vi "Set scrollbar at start.vi"(8 "error in (no error)":errorcluster, 11 "Queue in":refnum<queue>) -> (0 "error out":errorcluster)   [LabVIEW 2013]
uses:
  Typedefs/Speed Viewer States enum.ctl
  Globals/gl_Time series viewer globals.vi
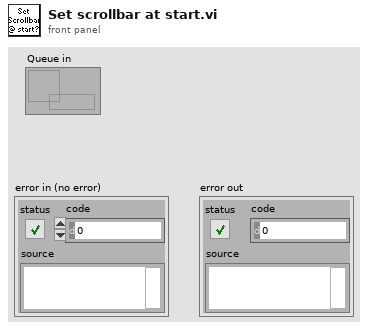
[diagram p1: front panel]
types:
  T1 = typedef "Timelapse viewer refs.ctl" = cluster{"This VI":refnum<vi>, "AVI Mode ind":refnum<vi>, "Play":refnum<vi>, "Stop":refnum<vi>, "Back":refnum<vi>, "Scrollbar":refnum<vi>, "Video length info":refnum<vi>, "Expected speed values":refnum<vi>, "Intensity":refnum<vi>, "Path":refnum<vi>, "Selection sliders":refnum<vi>, "Speed Graph ref":refnum<vi>, "Frame rate set (fps)":refnum<vi>}
  T2 = typedef "Speed Viewer States enum.ctl" = enum16{"Idle", "Initialise", "Playback", "Scroll bar event", "Speed cursor event", "Back to start", "Exit"}
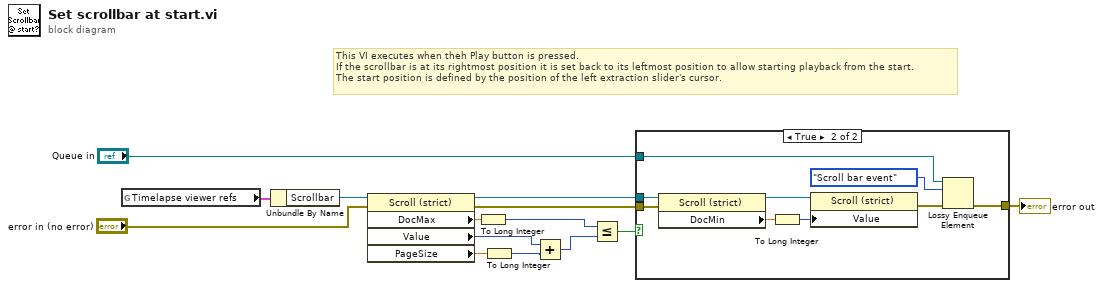
[diagram p0: block diagram]
diagram:
  # "This VI executes when theh Play button is pressed.\nIf the scrollbar is at its rightmost position it is set back to its leftmost position to allow starting playback from the start.\nThe start position is defined by the position of the left extraction slider's cursor."
  n1 = global read "gl_Time series viewer globals.vi" "Timelapse viewer refs"() -> (w14:T1)
  n2 = Unbundle By Name(w14) -> ("Scrollbar"=w13:refnum<vi>)
  n3 = property on="Property Node" class="Scroll (strict)"(reference=w13, error in="error in (no error)") -> (reference out=w9:refnum<vi>, error out=w10:errorcluster, "DocMax"=w11:dbl, "Value"=w4:i32, "PageSize"=w5:dbl)
  n4 = To Long Integer(number=w11) -> (32bit integer=w6:i32)
  n5 = To Long Integer(number=w5) -> (32bit integer=w2:i32)
  n6 = Add(x=w4, y=w2) -> (x+y=w3:i32)
  n7 = Less Or Equal?(x=w6, y=w3) -> (x <= y?=w7:bool)
  n8 = case shown="True" w7 {
    tunnel: w10 -> [w15 w22]
    tunnel: w9 -> [_ w21]
    tunnel: [w15 w18] -> w8
    tunnel: "Queue in" -> [_ w17]
    frame False {
    }
    frame True {
      n9 = property on="Property Node" class="Scroll (strict)"(reference=w21, error in=w22) -> (reference out=w23:refnum<vi>, "DocMin"=w24:dbl)  [unwired: 1 out]
      n10 = To Long Integer(number=w24) -> (32bit integer=w20:i32)
      n11 = property on="Property Node" class="Scroll (strict)"(reference=w23, "Value"=w20) -> (error out=w19:errorcluster)  [unwired: 1 in, 1 out]
      n12 = Lossy Enqueue Element(queue=w17, element=Speed_Viewer_States_enum."Scroll bar event" ("States"), error in (no error)=w19) -> (error out=w18:errorcluster)  [unwired: 3 out]
    }
  }
  "error out" <- w8
